vi "Get Instrument Configuration.vi"(8 "Error In":errorcluster, 10 "Instrument Identifier":string) -> (0 "Error Out":errorcluster, 1 "Instrument Configuration":refnum<class "Config from JSON.lvclass">, 2 "Found":bool)   [LabVIEW 2024, in "Instrument Manager.lvclass"]
uses:
  Instrument Manager.lvclass
  Config from JSON/Config from JSON.lvclass
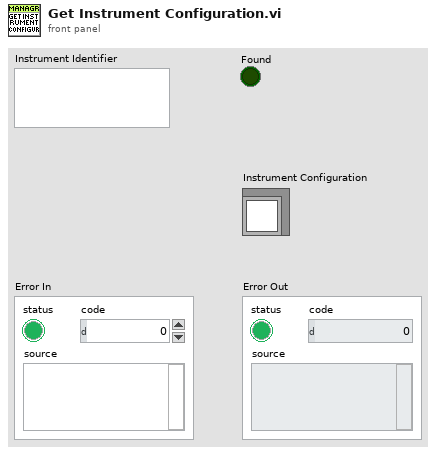
[diagram p1: front panel]
types:
  T1 = typedef "Instrument Manager.lvclass/ObjectAttributes.ctl" = cluster{"IInstruments":map{string, refnum<class "IInstrument.lvclass">}, "Instrument Configurations":map{string, refnum<class "Config from JSON.lvclass">}, "IVirtual Instruments":map{string, refnum<class "IVirtual Instrument.lvclass">}, "Virtual Instrument Configurations":map{string, refnum<class "Config from JSON.lvclass">}}
  T2 = map{string, refnum<class "Config from JSON.lvclass">}
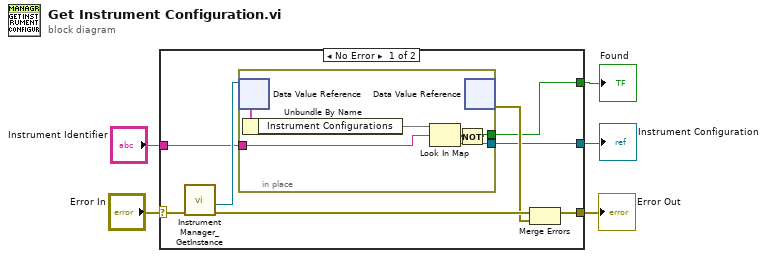
[diagram p0: block diagram]
diagram:
  n1 = case shown="No Error" "Error In" {
    selector: "Error In" -> [w13 w20]
    tunnel: [w11 w20] -> w4
    tunnel: [w9 _] -> w3
    tunnel: [w7 _] -> w2
    tunnel: "Instrument Identifier" -> [w6 _]
    frame No Error {
      n2 = call "Instrument Manager_GetInstance.vi"("Error In"=w13) -> ("Error Out"=w12:errorcluster, "DVRRefOut"=w8:refnum<data-value>)  [unwired: 6 in, 3 out]
      n3 = in-place {
        in-place-border: [w18] -> w9
        in-place-border: [w15] -> w7
        in-place-border: w6 -> [w14]
        n4 = in-place-dvr #1(w8) -> (w19:T1)  [unwired: 1 out]
        n5 = Unbundle By Name(w19) -> ("Instrument Configurations"=w17:T2)
        n6 = Look In Map(map=w17, key=w14) -> (key not found?=w16:bool, value=w18:refnum<class "Config from JSON.lvclass">)  [unwired: 1 in]
        n7 = Not(x=w16) -> (.not. x?=w15:bool)
        n8 = in-place-dvr #1() -> (w10:errorcluster)  [unwired: 1 in, 1 out]
      }
      n9 = Merge Errors(w12, w10) -> (w11:errorcluster)
    }
    frame Error {
    }
  }
  "Error Out" <- w4
  "Instrument Configuration" <- w3
  "Found" <- w2
